vi "cw_5_5.vi"() -> ()   [LabVIEW 2022 SP3]
uses:
  <vilib>/regexp/Match Regular Expression.xnode
panel:
  out "Activities found":string
  in  "Path":path=path "C:/Users/janek/OneDrive - Akademia Górniczo-Hutnicza im. Stanisława Staszica w Krakowie/sem_3/JAN_CICHON_LABVIEW/cw_5/Activities/Log_20221126.txt"
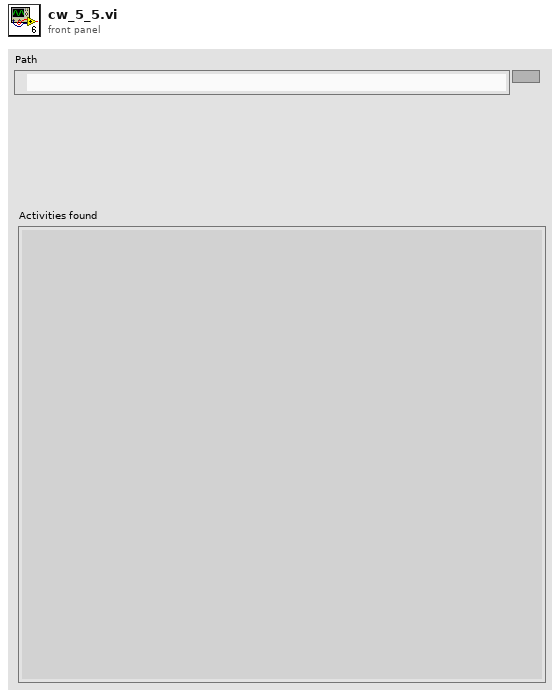
[diagram p1: front panel]
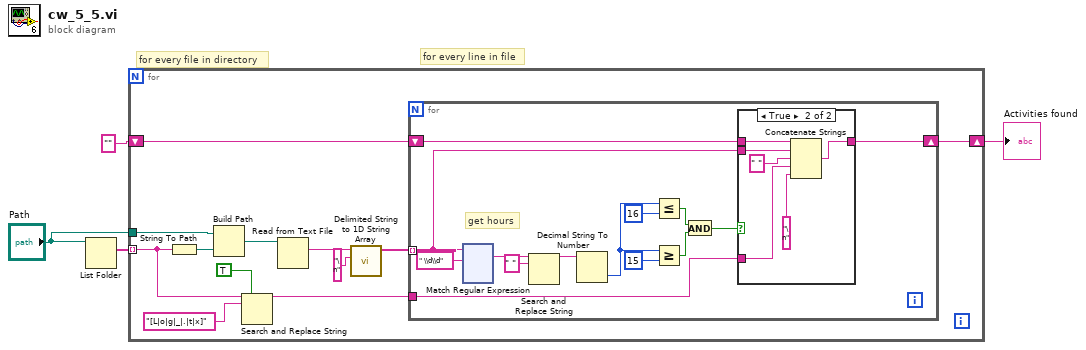
[diagram p0: block diagram]
diagram:
  # "for every line in file"
  # "for every file in directory"
  n1 = List Folder(path="Path") -> (filenames=w4:string[])  [unwired: 3 in, 3 out]
  n2 = for {
    tunnel: w4 -> [w11] mode=indexing
    tunnel: "Path" -> [w14]
    shift-right: [w8] -> w2
    shift-left: "" -> [w7]
    n3 = String To Path(string=w11) -> (path=w16:path)
    n4 = Build Path(base path=w14, name or relative path=w16) -> (appended path=w15:path)
    n5 = Search and Replace String(replace all?=TRUE ("replace all? (F)"), input string=w11, search string="[L|o|g|_|.|t|x]") -> (result string=w9:string)  [unwired: 5 in, 3 out]
    n6 = Read from Text File(file (use dialog)=w15) -> (text=w13:string)  [unwired: 3 in, 3 out]
    n7 = call <vilib>:"Delimited String to 1D String Array.vi"("delimiter"="\n", "delimited string"=w13) -> ("string array"=w12:string[])  [unwired: 9 in]
    n8 = for {
      tunnel: w12 -> [w20] mode=indexing
      tunnel: w9 -> [w19]
      shift-right: [w17] -> w8
      shift-left: w7 -> [w18]
      # "get hours"
      n9 = xnode "Match Regular Expression"("input string"=w20, "regular expression"=" \\d\\d") -> ("whole match"=w29:string)  [unwired: 4 in, 4 out]
      n10 = Search and Replace String(input string=w29, search string=" ") -> (result string=w27:string)  [unwired: 6 in, 3 out]
      n11 = Decimal String To Number(string=w27) -> (number=w26:i32)  [unwired: 2 in, 1 out]
      n12 = Less Or Equal?(x=w26, y=16) -> (x <= y?=w23:bool)
      n13 = Greater Or Equal?(x=w26, y=15) -> (x >= y?=w22:bool)
      n14 = And(x=w23, y=w22) -> (x .and. y?=w21:bool)
      n15 = case shown="True" w21 {
        tunnel: w20 -> [_ w36]
        tunnel: w19 -> [_ w32]
        tunnel: w18 -> [w31 w37]
        tunnel: [w31 w35] -> w17
        frame False {
        }
        frame True {
          n16 = Concatenate Strings(w37, w36, " " ("string"), w32, "\n" ("string")) -> (w35:string)
        }
      }
    }
  }
  "Activities found" <- w2
